vi "SimConfigRefGlobal.vi"() -> ()   [LabVIEW 2017, in "IrManageCameras.lvlib"]
uses:
  <vilib>/addons/InsightCM/Devices/Shared/Ir/IrManageCameras/IrManageCameras.lvlib
panel:
  in  "Sim Cameras":refnum<vi>
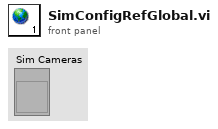
[diagram p1: front panel]
diagram:
